vi "Publish.vi"(6 "Publish Time":timestamp, 8 "error in (no error)":errorcluster, 9 "Data to Publish":variant, 10 "Topic Name":string, 11 "Mediator in":refnum<class "Mediator.lvclass">) -> (0 "error out":errorcluster, 3 "Mediator out":refnum<class "Mediator.lvclass">)   [LabVIEW 2015, in "Mediator.lvlib" / "Mediator.lvclass"]
doc: "<License>\nCopyright © 2017 Composed Systems, LLC | All rights reserved\nwww.composed.io\n\nAuthor: Ethan Stern <ethan.stern@composed.io>\n\nThis software is provided \"AS IS\" WITHOUT WARRANTIES, either express or implied, AND IS FOR EDUCATIONAL PURPOSES ONLY.\n</License>"
uses:
  Mediator.lvclass
  Mediator.lvclass/Mediator.ctl
  Topic Messages/Notify Subscribers Msg/Notify Subscribers Msg.lvclass/Notify Subscribers Msg.ctl
  <vilib>/ActorFramework/Message Enqueuer/Message Enqueuer.lvclass/Message Enqueuer.ctl
  <vilib>/ActorFramework/Message Enqueuer/Enqueue.vi
  <vilib>/ActorFramework/Message Priority Queue/Priority Enqueue.vi
  Topic Messages/Notify Subscribers Msg/Notify Subscribers Msg.lvclass
  TopicLookupTable/TopicLookupTable.lvclass
  Topic/Topic.lvclass
  <vilib>/ActorFramework/Actor/Actor.lvclass
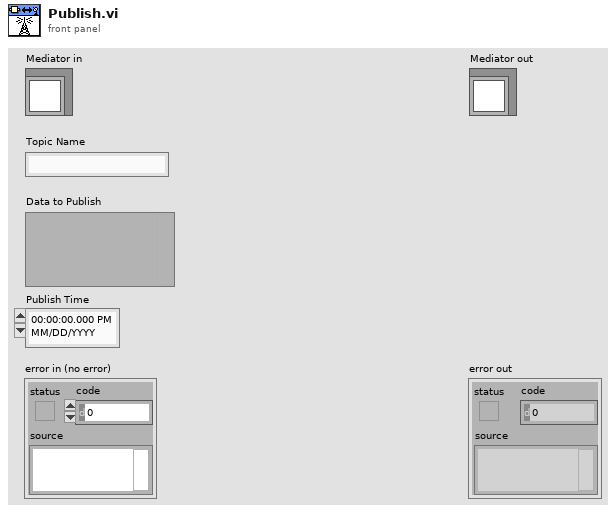
[diagram p1: front panel]
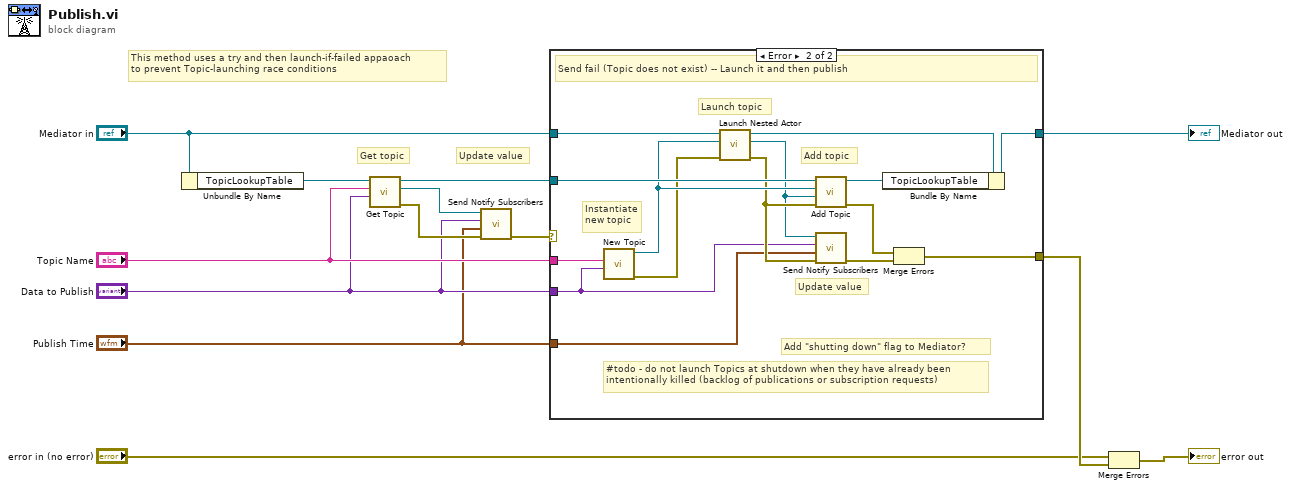
[diagram p0: block diagram]
diagram:
  # "This method uses a try and then launch-if-failed appaoach\nto prevent Topic-launching race conditions"
  # "Update value"
  # "Get topic"
  n1 = Unbundle By Name("Mediator in") -> ("TopicLookupTable"=w12:refnum<class "TopicLookupTable.lvclass">)
  n2 = call "Get Topic.vi"("Topic Type"="Data to Publish", "Topic Name"="Topic Name", "TopicLookupTable in"=w12) -> ("error out"=w8:errorcluster, "Topic Refnum"=w13:refnum<class "Message Enqueuer.lvclass">, "TopicLookupTable out"=w11:refnum<class "TopicLookupTable.lvclass">)  [unwired: 5 in, 1 out]
  n3 = call "Send Notify Subscribers.vi"("error in (no error)"=w8, "Publish Time"="Publish Time", "Topic Data"="Data to Publish", "Message Enqueuer"=w13) -> ("error out"=w10:errorcluster)  [unwired: 6 in, 1 out]
  n4 = case shown="Error" w10 {
    selector: w10 -> [w14 _]
    tunnel: w11 -> [_ w27]
    tunnel: "Mediator in" -> [w15 w30]
    tunnel: [w15 w16] -> w6
    tunnel: "Topic Name" -> [_ w28]
    tunnel: "Data to Publish" -> [_ w18]
    tunnel: [w14 w21] -> w9
    tunnel: "Publish Time" -> [_ w17]
    frame No Error {
      # "Subscribe OK (Topic is alive)"
    }
    frame Error {
      # "Add \"shutting down\" flag to Mediator?"
      # "#todo - do not launch Topics at shutdown when they have already been\nintentionally killed (backlog of publications or subscription requests)"
      # "Launch topic"
      # "Add topic"
      # "Update value"
      # "Instantiate\nnew topic"
      # "Send fail (Topic does not exist) -- Launch it and then publish"
      n5 = call "New Topic.vi"("Data Type"=w18, "Name"=w28) -> ("error out"=w24:errorcluster, "Topic out"=w25:refnum<class "Topic.lvclass">)  [unwired: 8 in]
      n6 = call <vilib>:"Launch Nested Actor.vi"("error in (no error)"=w24, "Nested Actor"=w25, "Caller Actor in"=w30) -> ("error out"=w20:errorcluster, "Nested Actor's Enqueuer"=w19:refnum<class "Message Enqueuer.lvclass">, "Caller Actor out"=w29:refnum<class "Mediator.lvclass">)  [unwired: 6 in]
      n7 = call "Add Topic.vi"("error in (no error)"=w20, "Topic Enqueuer"=w19, "Topic Object"=w25, "TopicLookupTable in"=w27) -> ("error out"=w23:errorcluster, "TopicLookupTable out"=w26:refnum<class "TopicLookupTable.lvclass">)  [unwired: 5 in, 1 out]
      n8 = call "Send Notify Subscribers.vi"("error in (no error)"=w20, "Publish Time"=w17, "Topic Data"=w18, "Message Enqueuer"=w19) -> ("error out"=w22:errorcluster)  [unwired: 6 in, 1 out]
      n9 = Bundle By Name(cluster=w29, "TopicLookupTable"=w26) -> (w16:refnum<class "Mediator.lvclass">)
      n10 = Merge Errors(w23, w22) -> (w21:errorcluster)
    }
  }
  "Mediator out" <- w6
  n11 = Merge Errors("error in (no error)", w9) -> (→"error out":errorcluster)
